vi "Initialize.vi"(8 "error in (no error)":errorcluster, 11 "BL-Extend-Cmd in":refnum<class "BL-Extend-Cmd.lvclass">) -> (0 "error out":errorcluster, 3 "BL-Extend-Cmd out":refnum<class "BL-Extend-Cmd.lvclass">)   [LabVIEW 2013, in "BL-Extend-Cmd.lvclass"]
uses:
  BL-Extend-Cmd.lvclass
  States/BL-Extending-State/BL-Extending-State.lvclass
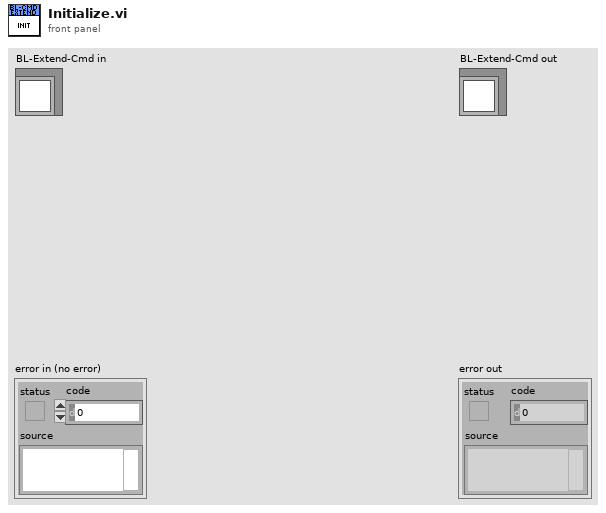
[diagram p1: front panel]
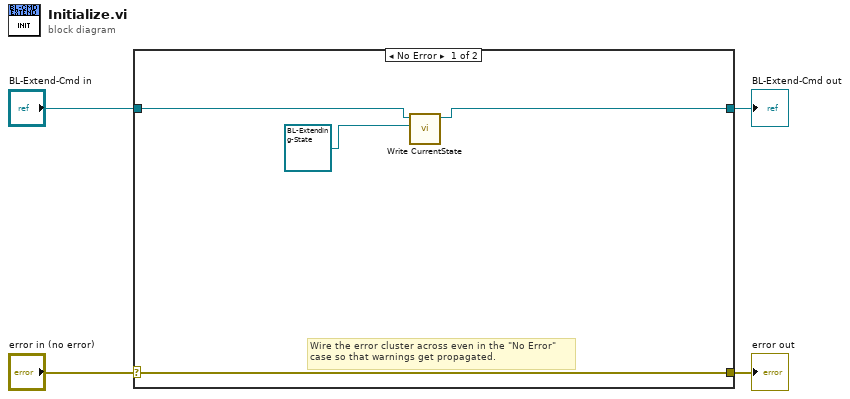
[diagram p0: block diagram]
diagram:
  n1 = case shown="No Error" "error in (no error)" {
    selector: "error in (no error)" -> [w8 w10]
    tunnel: [w8 w10] -> w3
    tunnel: [w6 w9] -> w1
    tunnel: "BL-Extend-Cmd in" -> [w7 w9]
    frame No Error {
      # "Wire the error cluster across even in the \"No Error\"\ncase so that warnings get propagated."
      n2 = call-dynamic "Write CurrentState.vi"("State.lvclass"=refnum<class "BL-Extending-State.lvclass"> refnum ("BL-Extending-State.lvclass"), "Command in"=w7) -> ("Command out"=w6:refnum<class "BL-Extend-Cmd.lvclass">)  [unwired: 8 in, 1 out]
    }
    frame Error {
    }
  }
  "error out" <- w3
  "BL-Extend-Cmd out" <- w1
